vi "Do.vi"(8 "error in":errorcluster, 10 "Actor in":refnum<class "Actor.lvclass">, 11 "Toggle AC Spare MSG":refnum<class "Toggle AC Spare MSG.lvclass">) -> (0 "error out":errorcluster, 2 "Actor out":refnum<class "Actor.lvclass">)   [LabVIEW 2016, in "Controller.lvlib" / "Toggle AC Spare MSG.lvclass"]
doc: "(<B>Filename</B>: Actor Framework.lvlib:Message.lvclass:Do.vi)\n\nDefines what a message does when it is received by an actor. Generally, a message instructs an actor to invoke one of its methods. By default, this method does nothing. A child class must override it to define behavior. Create a child class by using the Actor Framework Message Maker dialog box."
uses:
  Toggle AC Spare MSG.lvclass
  G:/sw_repo/For Builds/Nicholas/Controller/Messages/Generic Boolean MSG/Generic Boolean Message.lvclass
  <vilib>/ActorFramework/Actor/Actor.lvclass
  Generic Boolean MSG/Generic Boolean Message.lvclass/Generic Boolean Message.ctl
  gController.lvclass
  C:/Program Files (x86)/National Instruments/LabVIEW 2016/vi.lib/ActorFramework/Actor/Actor.lvclass
  Global FPGA DO.ctl
  Generic Boolean MSG/Read Bool.vi
  Global DO.vi
  <vilib>/rvi/errors/niLvFpgaAdjustHostInterfaceError.vi
  <vilib>/Utility/error.llb/Error Cluster From Error Code.vi
  FPGA Ref.ctl
  <vilib>/rvi/interface/nirviReadWriteControl/nirviReadWriteControl.xnode
  FPGA Bitfiles/server_v0_2_1_3.lvbitx
  NiFpgaLv.dll
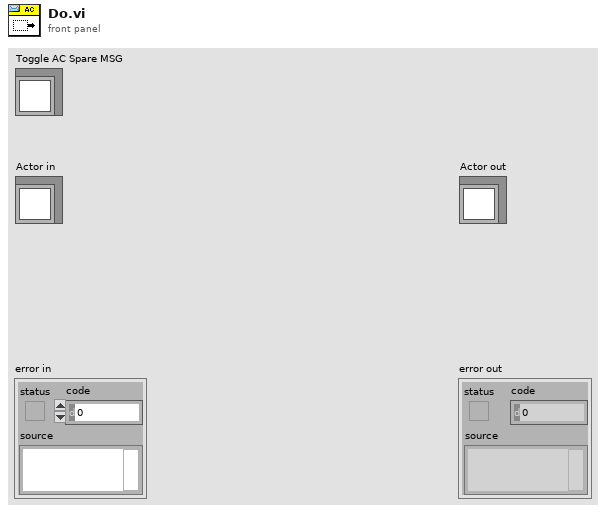
[diagram p1: front panel]
types:
  T1 = typedef "Global FPGA DO.ctl" = enum16{"pas_laser_relay_1", "pas_heater_1", "pas_heater_2", "pas_laser_relay_2", "pas_spk_enable_1", "pas_spk_enable_2", "hanbay_pos", "fan_enable", "crd_laser_enable", "crd_heater_enable", "vacuum_pump", "ac_spare", "uv_enable", "solenoid_1", "solenoid_2", "spare_dc_relay_1", "usb_hub_relay", "spare_dc_relay_2", "fp_aux_1", "fp_aux_2"}
  T2 = typedef "FPGA Ref.ctl" = refnum<k20>
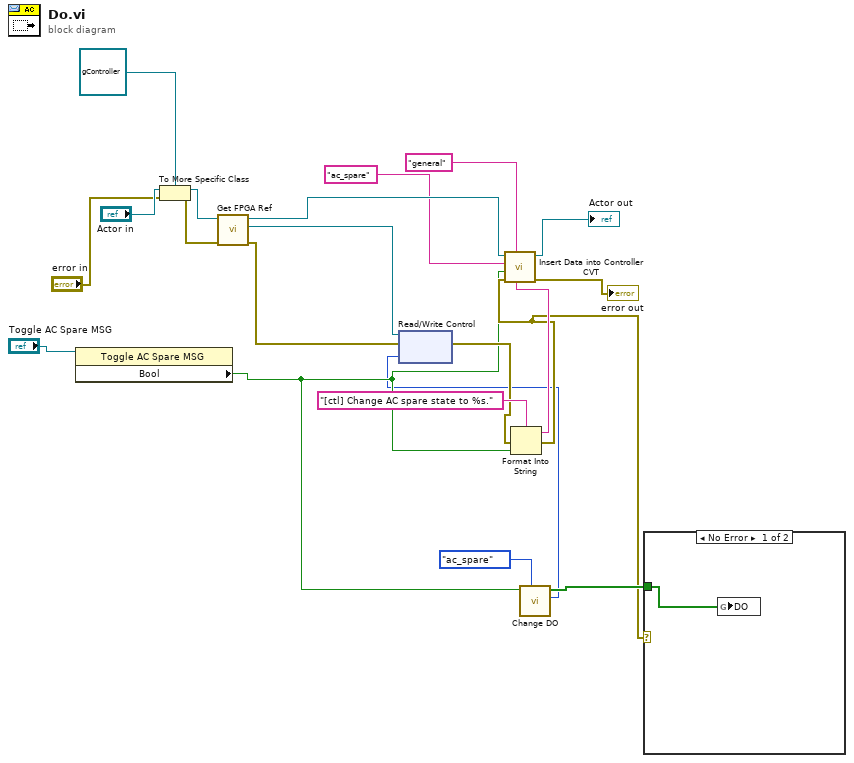
[diagram p0: block diagram]
diagram:
  n1 = property class="Toggle AC Spare MSG"(reference="Toggle AC Spare MSG") -> ("Bool"=w2:bool)  [unwired: 1 in, 2 out]
  n2 = To More Specific Class(target class=refnum<class "gController.lvclass"> refnum ("Controller.lvlib:gController"), reference="Actor in", error in="error in") -> (specific class reference=w19:refnum<class "gController.lvclass">, error out=w17:errorcluster)
  n3 = call "Get FPGA Ref.vi"("error in (no error)"=w17, "Actor In"=w19) -> ("error out"=w8:errorcluster, "FPGA Ref"=w15:T2, "Actor Out"=w14:refnum<class "Actor.lvclass">)  [unwired: 7 in]
  n4 = call "Change DO.vi"("DO"=Global_FPGA_DO."ac_spare", "val_in"=w2) -> ("DO Long Out"=w1:u32, "DO Out"=w4:bool[])  [unwired: 8 in]
  n5 = xnode "Read/Write Control"("FPGA VI Reference In"=w15, "error in"=w8, "DO"=w1) -> ("error out"=w7:errorcluster)  [unwired: 1 out]
  n6 = Format Into String(format string="[ctl] Change AC spare state to %s.", error in=w7, w2) -> (resulting string=w9:string, error out=w3:errorcluster)  [unwired: 1 in]
  n7 = call "Insert Data into Controller CVT.vi"("Update MSG"=w9, "Group"="general", "error in"=w3, "Data"=w2, "tag"="ac_spare", "Actor in"=w14) -> ("error out"=→"error out":errorcluster, "Actor Out"=→"Actor out":refnum<class "Actor.lvclass">)  [unwired: 4 in]
  n8 = case shown="No Error" w3 {
    tunnel: w4 -> [w22 _]
    frame No Error {
      n9 = global write "Global DO.vi" "DO"(w22) -> ()
    }
    frame Error {
    }
  }
